vi "Fit Line - 3D.vi"(8 "error in (no error)":errorcluster, 11 "Points":refnum<class "Vec3d.lvclass">[](array[class])) -> (0 "error out":errorcluster, 1 "residual":dbl, 2 "centroid":refnum<class "Vec3d.lvclass">, 3 "direction":refnum<class "Vec3d.lvclass">)   [LabVIEW 2023]
uses:
  Vec3d Class/Vec3d.lvclass
  <vilib>/Math Plots/3D Math Plots/3D Scatter/3D Scatter XCtrl/3D Scatter.xctl
  <vilib>/Analysis/baseanly.llb/Mean (DBL).vi
  <vilib>/Analysis/Matrix/Numeric/Conversions/Array To Matrix - RA2.vi
  <vilib>/Analysis/7linalg.llb/Real SVD Decomposition.vi
  <vilib>/Analysis/Matrix/Numeric/Conversions/Matrix To Array - RM.vi
  <vilib>/Analysis/NI_AALBase.lvlib
  <vilib>/Analysis/NI_AALPro.lvlib
  <vilib>/Analysis/Matrix/NI_Matrix.lvlib
  <vilib>/Math Plots/3D Math Plots/3D Scatter/3D Scatter Datatype/3D Scatter Datatype.lvclass
  <vilib>/Math Plots/3D Math Plots/3D Scatter/3D Scatter Datatype/Public/Plot Helper (Vector).vi
panel:
  out "3D Scatter":refnum<class "3D Plot Datatype.lvclass">[](xcontrol)
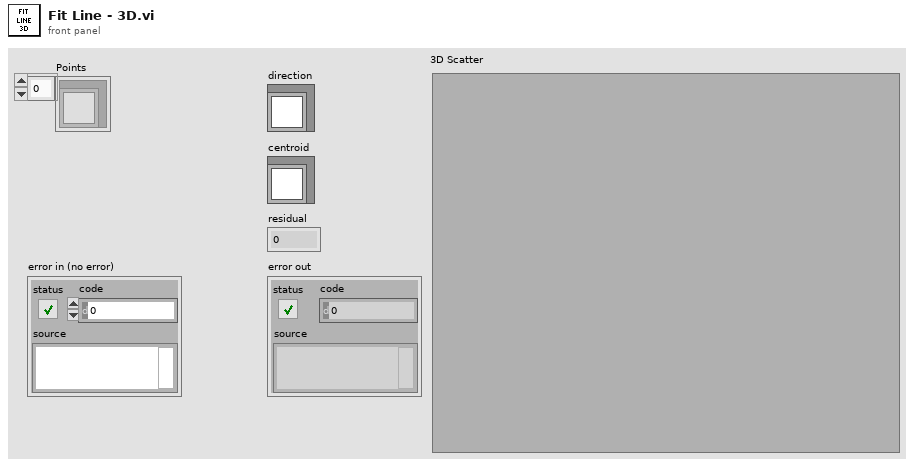
[diagram p1: front panel]
types:
  T1 = typedef "NI_Matrix.lvlib/RealMatrix.ctl" = dbl[][]
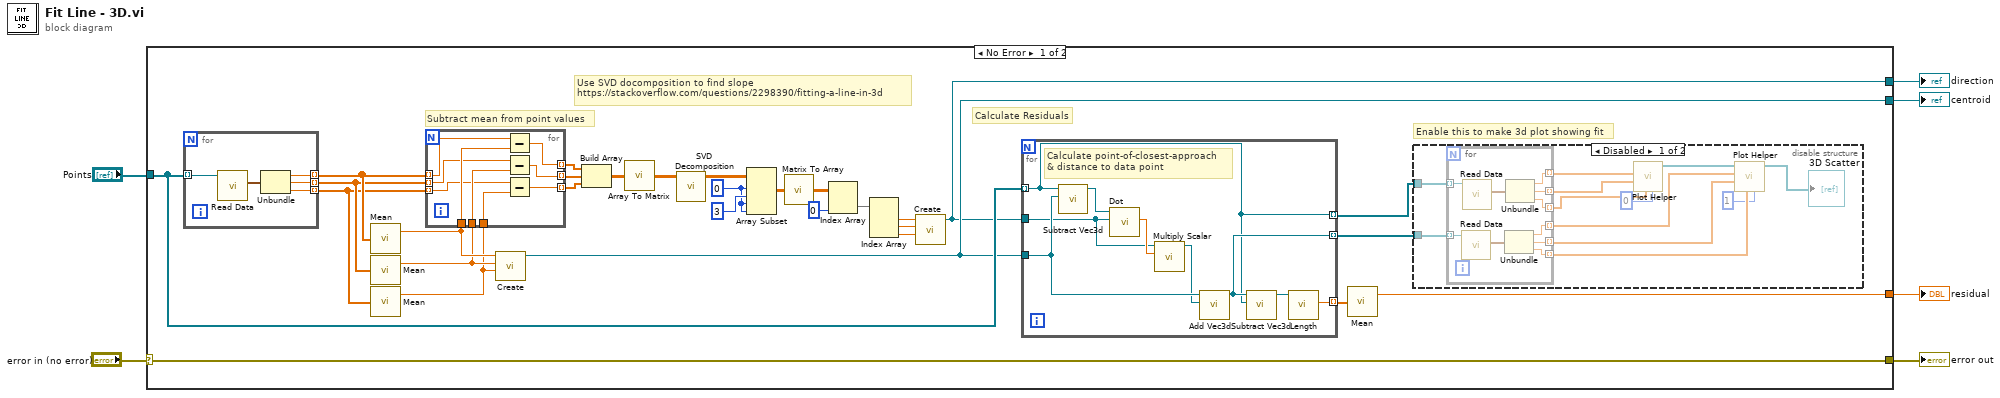
[diagram p0: block diagram]
diagram:
  n1 = case shown="No Error" "error in (no error)" {
    selector: "error in (no error)" -> [w27 w81]
    tunnel: "Points" -> [w13 _]
    tunnel: [w27 w81] -> w4
    tunnel: [w11 _] -> w3
    tunnel: [w12 _] -> w2
    tunnel: [w9 _] -> w1
    frame No Error {
      w24 = 0 ("row 1")
      # "Enable this to make 3d plot showing fit"
      # "Calculate Residuals"
      # "Use SVD docomposition to find slope\nhttps://stackoverflow.com/questions/2298390/fitting-a-line-in-3d"
      # "Subtract mean from point values"
      n2 = for {
        tunnel: w13 -> [w80] mode=indexing
        tunnel: [w78] -> w35 mode=indexing
        tunnel: [w77] -> w34 mode=indexing
        tunnel: [w76] -> w33 mode=indexing
        n3 = call-dynamic "Read Data.vi"("Vec3d Class in"=w80) -> ("Data"=w79:cluster{"X":dbl, "Y":dbl, "Z":dbl})  [unwired: 8 in, 2 out]
        n4 = Unbundle(w79) -> ("X"=w78:dbl, "Y"=w77:dbl, "Z"=w76:dbl)
      }
      n5 = call-poly <vilib>:"Mean.vi"("X"=w35) -> ("mean"=w16:dbl)  [unwired: 1 out]
      n6 = call-poly <vilib>:"Mean.vi"("X"=w34) -> ("mean"=w15:dbl)  [unwired: 1 out]
      n7 = call-poly <vilib>:"Mean.vi"("X"=w33) -> ("mean"=w14:dbl)  [unwired: 1 out]
      n8 = for {
        tunnel: w35 -> [w75] mode=indexing
        tunnel: w34 -> [w73] mode=indexing
        tunnel: w33 -> [w70] mode=indexing
        tunnel: w16 -> [w74]
        tunnel: w15 -> [w72]
        tunnel: w14 -> [w71]
        tunnel: [w69] -> w30 mode=indexing
        tunnel: [w68] -> w31 mode=indexing
        tunnel: [w67] -> w32 mode=indexing
        n9 = Subtract(x=w75, y=w74) -> (x-y=w67:dbl)
        n10 = Subtract(x=w73, y=w72) -> (x-y=w68:dbl)
        n11 = Subtract(x=w70, y=w71) -> (x-y=w69:dbl)
      }
      n12 = call "Create.vi"("Z"=w14, "Y"=w15, "X"=w16) -> ("Vec3d Class out"=w12:refnum<class "Vec3d.lvclass">)  [unwired: 7 in, 1 out]
      n13 = Build Array(w32, w31, w30) -> (w29:dbl[][])
      n14 = call-poly <vilib>:"Array To Matrix.vi"("Real 2D Array"=w29) -> ("Real Matrix"=w28:T1)
      n15 = call-poly <vilib>:"SVD Decomposition.vi"("A"=w28) -> ("Matrix U"=w26:T1)  [unwired: 6 in, 4 out]
      n16 = Array Subset(array=w26, index (row)=w24, length (row)=3 ("column N"), index (col)=w24, length (col)=w24) -> (w23:T1)
      n17 = call-poly <vilib>:"Matrix To Array.vi"("Real Matrix"=w23) -> ("Real 2D Array"=w22:dbl[][])
      n18 = Index Array(array=w22, index (col)=0 ("index (row)")) -> (element=w20:dbl[])  [unwired: 1 in]
      n19 = Index Array(array=w20) -> (element #1=w19:dbl, element #2=w18:dbl, element #3=w17:dbl)  [unwired: 3 in]
      n20 = call "Create.vi"("Z"=w17, "Y"=w18, "X"=w19) -> ("Vec3d Class out"=w11:refnum<class "Vec3d.lvclass">)  [unwired: 7 in, 1 out]
      n21 = for {
        tunnel: w13 -> [w58] mode=indexing
        tunnel: w12 -> [w65]
        tunnel: w11 -> [w63]
        tunnel: [w61] -> w10 mode=indexing
        tunnel: [w59] -> w7 mode=indexing
        tunnel: [w58] -> w8 mode=indexing
        # "Calculate point-of-closest-approach\n& distance to data point"
        n22 = call "Subtract Vec3d.vi"("Vec3d in 2"=w65, "Vec3d in 1"=w58) -> ("Vec3d Class out"=w66:refnum<class "Vec3d.lvclass">)  [unwired: 8 in, 1 out]
        n23 = call "Dot.vi"("Vec3d in 2"=w63, "Vec3d in 1"=w66) -> ("Dot Product"=w64:dbl)  [unwired: 8 in, 1 out]
        n24 = call-dynamic "Multiply Scalar.vi"("Scale"=w64, "Vec3d in"=w63) -> ("Vec3d out"=w62:refnum<class "Vec3d.lvclass">)  [unwired: 8 in, 1 out]
        n25 = call-dynamic "Add Vec3d.vi"(10:"Vec3d Class in"=w62, 11:"Vec3d Class in"=w65) -> ("Vec3d Class out"=w59:refnum<class "Vec3d.lvclass">)  [unwired: 8 in, 1 out]
        n26 = call "Subtract Vec3d.vi"("Vec3d in 2"=w58, "Vec3d in 1"=w59) -> ("Vec3d Class out"=w60:refnum<class "Vec3d.lvclass">)  [unwired: 8 in, 1 out]
        n27 = call-dynamic "Length.vi"("Vec3d in"=w60) -> ("Length"=w61:dbl)  [unwired: 8 in, 2 out]
      }
      n28 = call-poly <vilib>:"Mean.vi"("X"=w10) -> ("mean"=w9:dbl)  [unwired: 1 out]
      n29 = disable-structure shown="Disabled" {
        disable-tunnel: w8 -> [w47 _]
        disable-tunnel: w7 -> [w46 _]
        frame Disabled {
          n30 = for {
            tunnel: w47 -> [w54] mode=indexing
            tunnel: w46 -> [w55] mode=indexing
            tunnel: [w53] -> w45 mode=indexing
            tunnel: [w52] -> w44 mode=indexing
            tunnel: [w51] -> w43 mode=indexing
            tunnel: [w50] -> w40 mode=indexing
            tunnel: [w49] -> w39 mode=indexing
            tunnel: [w48] -> w38 mode=indexing
            n31 = call-dynamic "Read Data.vi"("Vec3d Class in"=w55) -> ("Data"=w56:cluster{"X":dbl, "Y":dbl, "Z":dbl})  [unwired: 8 in, 2 out]
            n32 = call-dynamic "Read Data.vi"("Vec3d Class in"=w54) -> ("Data"=w57:cluster{"X":dbl, "Y":dbl, "Z":dbl})  [unwired: 8 in, 2 out]
            n33 = Unbundle(w56) -> ("X"=w50:dbl, "Y"=w49:dbl, "Z"=w48:dbl)
            n34 = Unbundle(w57) -> ("X"=w53:dbl, "Y"=w52:dbl, "Z"=w51:dbl)
          }
          n35 = call-poly <vilib>:"Plot Helper.vi"("Plot ID"=0, "z vector"=w43, "y vector"=w44, "x vector"=w45) -> ("3D Plot lvclass Array out"=w42:refnum<class "3D Plot Datatype.lvclass">[])  [unwired: 2 in, 5 out]
          n36 = call-poly <vilib>:"Plot Helper.vi"("Plot ID"=1, "z vector"=w38, "y vector"=w39, "x vector"=w40, "3D Plot lvclass Array in"=w42) -> ("3D Plot lvclass Array out"=→"3D Scatter":refnum<class "3D Plot Datatype.lvclass">[])  [unwired: 1 in, 5 out]
        }
        frame Enabled {
        }
      }
    }
    frame Error {
    }
  }
  "error out" <- w4
  "direction" <- w3
  "centroid" <- w2
  "residual" <- w1
